vi "reading external parameters.vi"(6 "debug?":bool, 8 "error in (no error)":errorcluster, 11 "path _calib.dat":path) -> (0 "error out":errorcluster, 3 "ROIs cluster":T1)   [LabVIEW 2023]
uses:
  control/rois list cluster.ctl
  <vilib>/Utility/file.llb/Read Delimited Spreadsheet (string).vi
  <vilib>/Utility/file.llb/Read Delimited Spreadsheet (DBL).vi
panel:
  out "ROIs List":cluster{"String":string, "Value":i32}[](array[cluster])
  out "List ROI out":dbl[][](array[numeric])
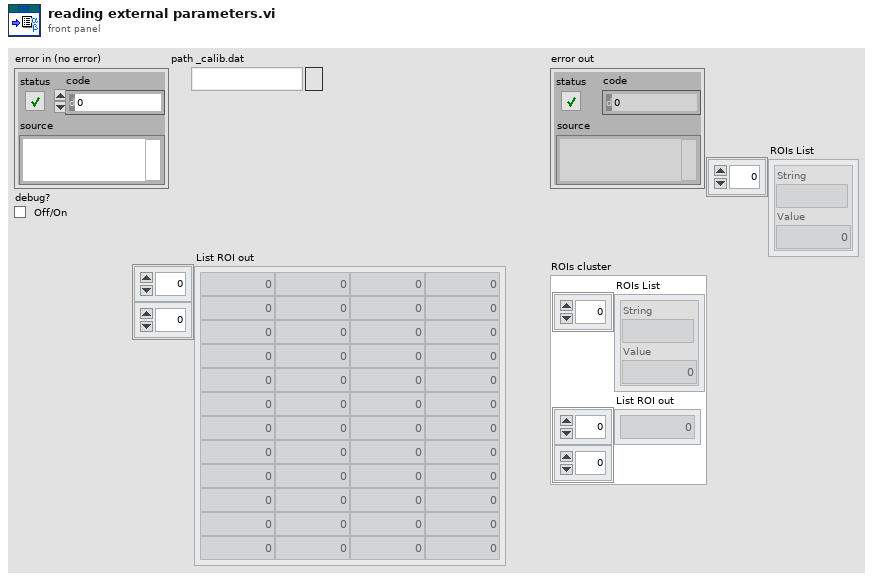
[diagram p1: front panel]
types:
  T1 = typedef "rois list cluster.ctl" = cluster{"ROIs List":cluster{"String":string, "Value":i32}[], "List ROI out":dbl[][]}
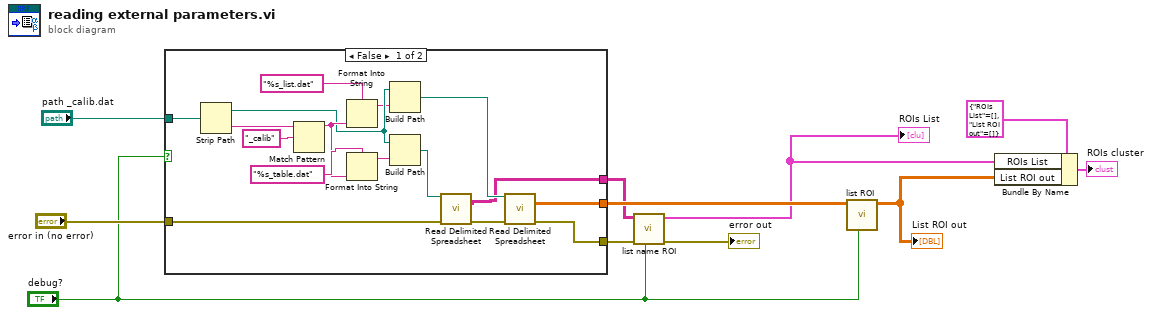
[diagram p0: block diagram]
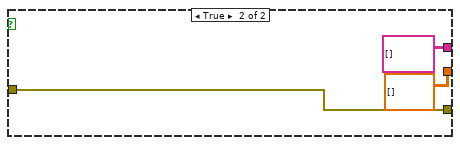
[diagram p2: hidden frame]
diagram:
  n1 = case shown="False" "debug?" {
    tunnel: "error in (no error)" -> [w16 w28]
    tunnel: "path _calib.dat" -> [w15 _]
    tunnel: [w14 dbl[][] [] ("all rows")] -> w9
    tunnel: [w13 w28] -> w8
    tunnel: [w12 string[][] [] ("all rows")] -> w6
    frame False {
      n2 = Strip Path(path=w15) -> (stripped path=w20:path, name=w23:string)
      n3 = Match Pattern(string=w23, regular expression="_calib" ("format string")) -> (before substring=w21:string)  [unwired: 1 in, 3 out]
      n4 = Format Into String(format string="%s_list.dat", w21) -> (resulting string=w19:string)  [unwired: 2 in, 1 out]
      n5 = Format Into String(format string="%s_table.dat", w21) -> (resulting string=w25:string)  [unwired: 2 in, 1 out]
      n6 = Build Path(base path=w20, name or relative path=w19) -> (appended path=w18:path)
      n7 = Build Path(base path=w20, name or relative path=w25) -> (appended path=w24:path)
      n8 = call-poly <vilib>:"Read Delimited Spreadsheet.vi"("file path (dialog if empty)"=w24, "error in (no error)"=w16) -> ("all rows"=w12:string[][], "error out"=w17:errorcluster)  [unwired: 8 in, 4 out]
      n9 = call-poly <vilib>:"Read Delimited Spreadsheet.vi"("file path (dialog if empty)"=w18, "error in (no error)"=w17) -> ("all rows"=w14:dbl[][], "error out"=w13:errorcluster)  [unwired: 8 in, 4 out]
    }
    frame True {
    }
  }
  n10 = call "list name ROI.vi"("debug?"="debug?", "error in"=w8, "Elements Selected"=w6) -> ("error out"=→"error out":errorcluster, "ROIs List"=w4:cluster{"String":string, "Value":i32}[])  [unwired: 7 in]
  "ROIs List" <- w4
  n11 = call "list ROI.vi"("debug?"="debug?", "List ROI in"=w9) -> ("List ROI out"=w3:dbl[][])  [unwired: 9 in]
  "List ROI out" <- w3
  n12 = Bundle By Name(cluster=T1 {"ROIs List"=[], "List ROI out"=[]}, "ROIs List"=w4, "List ROI out"=w3) -> (→"ROIs cluster":T1)
